vi "WM_CAP - Edit Format.vi"(0 "hwnd":u32, 5 "WM_CAP_START":u32, 11 "Error":errorcluster) -> (15 "error out":errorcluster)   [LabVIEW 2022 SP3]
uses:
  user32.dll
panel:
  in  "Apply":bool
  in  "Compression":string
  in  "BitCount":i16=24
  in  "Height":i32=480
  in  "Width":i32=640
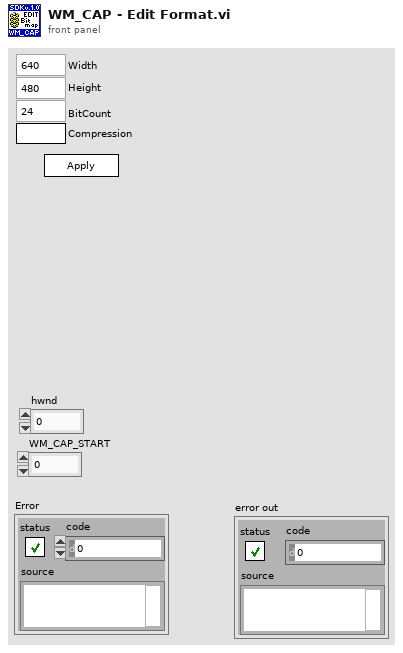
[diagram p1: front panel]
types:
  T1 = cluster{"biSize":i32, "biWidth":i32, "biHeight":i32, "biPlanes":i16, "biBitCount":i16, "biCompression":i32, "biSizeImage":i32, "biXPelsPerMeter":i32, "biYPelsPerMeter":i32, "biClrUsed":i32, "biClrImportant":i32, "Colors":u32[]}
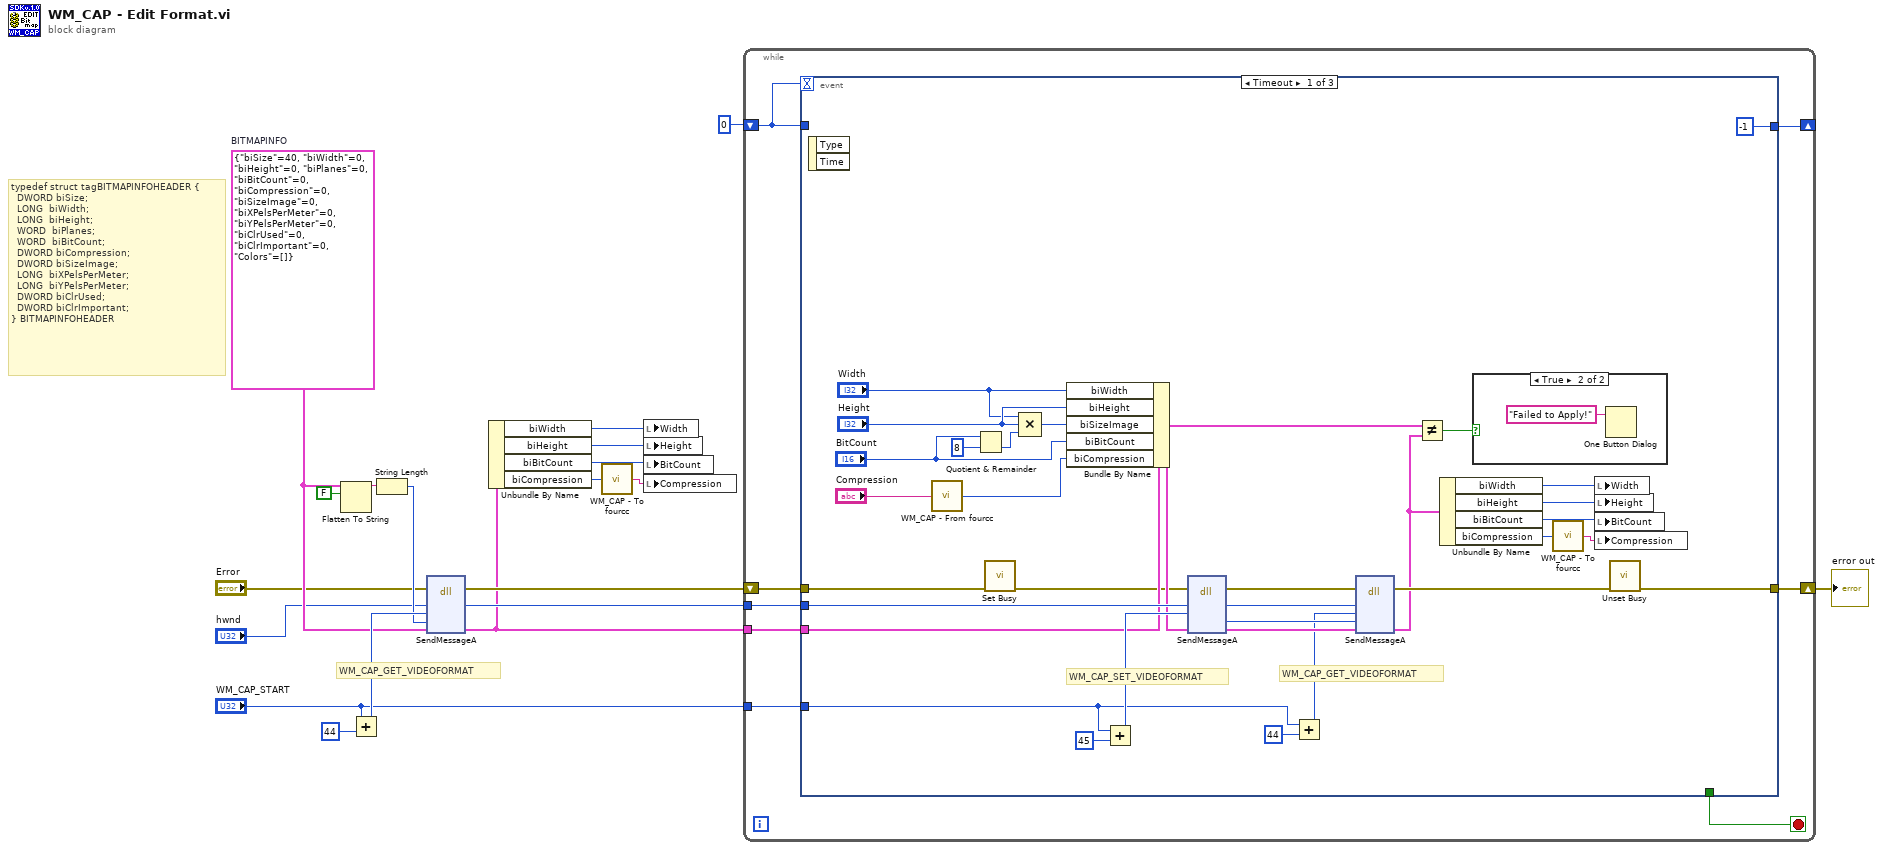
[diagram p0: block diagram]
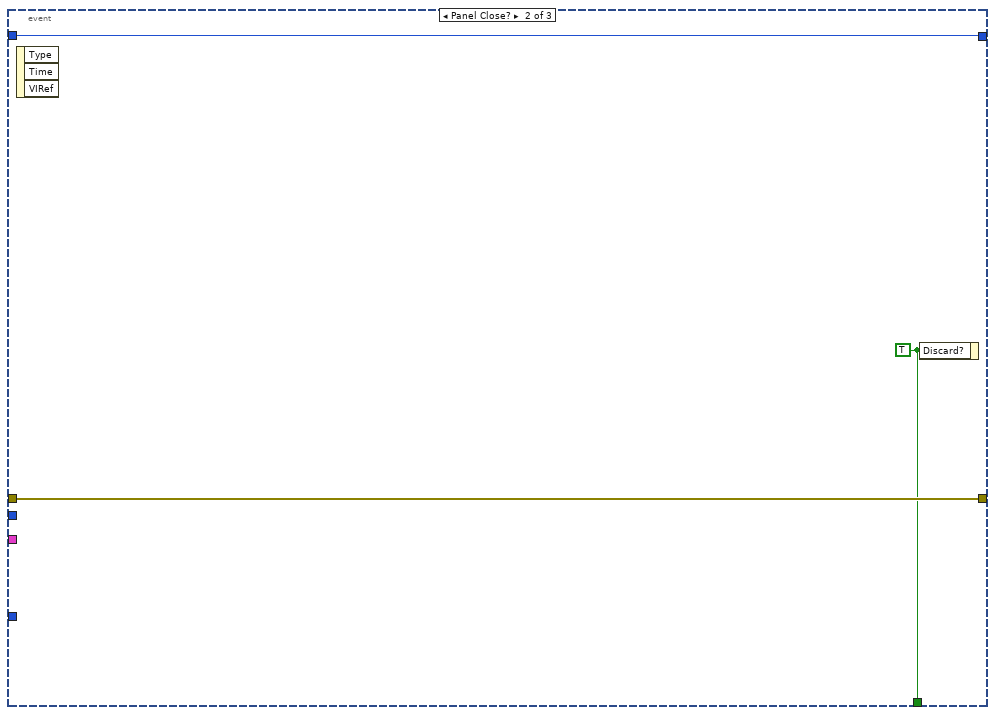
[diagram p3: hidden frame]
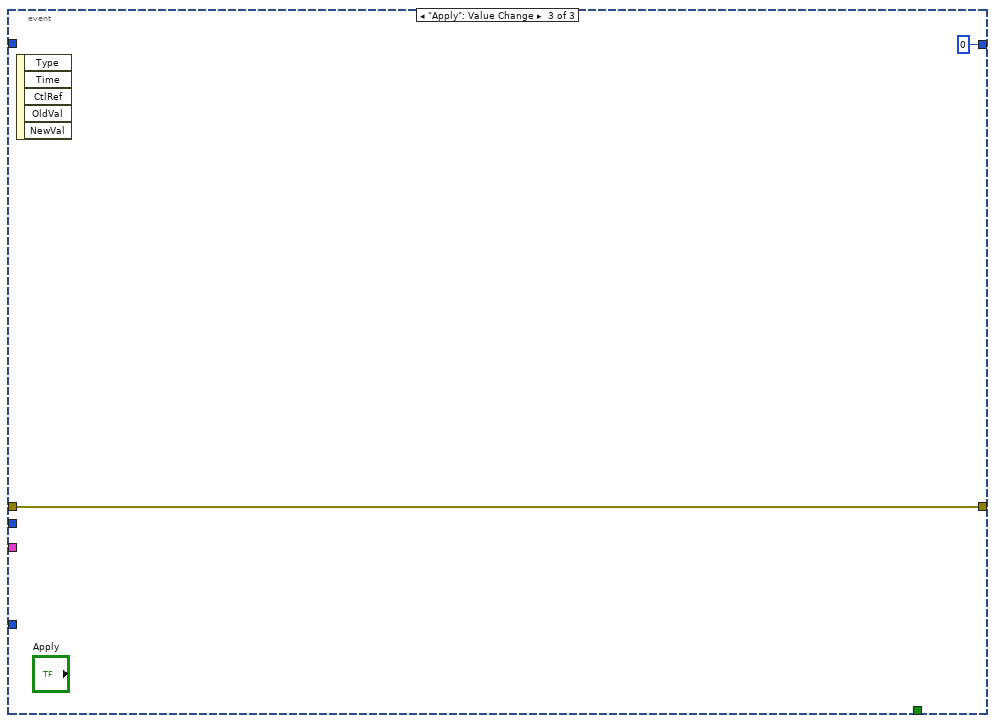
[diagram p4: hidden frame]
diagram:
  w12 = T1 {"biSize"=40, "biWidth"=0, "biHeight"=0, "biPlanes"=0, "biBitCount"=0, "biCompression"=0, "biSizeImage"=0, "biXPelsPerMeter"=0, "biYPelsPerMeter"=0, "biClrUsed"=0, "biClrImportant"=0, "Colors"=[]}  # BITMAPINFO
  # "typedef struct tagBITMAPINFOHEADER {\n  DWORD biSize;\n  LONG  biWidth;\n  LONG  biHeight;\n  WORD  biPlanes;\n  WORD  biBitCount;\n  DWORD biCompression;\n  DWORD biSizeImage;\n  LONG  biXPelsPerMeter;\n  LONG  biYPelsPerMeter;\n  DWORD biClrUsed;\n  DWORD biClrImportant;\n} BITMAPINFOHEADER"
  # "WM_CAP_GET_VIDEOFORMAT"
  n1 = Flatten To String(anything=w12, prepend array or string size? (T)=FALSE) -> (data string=w14:string)  [unwired: 2 in, 2 out]
  n2 = Add(x="WM_CAP_START", y=u16 44) -> (x+y=w17:u32)
  n3 = String Length(string=w14) -> (length=w16:i32)
  n4 = dll-call lib="user32.dll" fn="SendMessageA"(error in="Error", "hwnd"="hwnd", "msg"=w17, "wParam"=w16, "lparam"=w12) -> (error out=w9:errorcluster, "hwnd"=w7:u32, "lparam"=w6:T1)  [unwired: 5 in, 1 out]
  n5 = Unbundle By Name(w6) -> ("biWidth"=w5:i32, "biHeight"=w4:i32, "biBitCount"=w3:i16, "biCompression"=w2:i32)
  n6 = call "WM_CAP - To fourcc.vi"("biCompression"=w2) -> ("FOURCC"=w1:string)  [unwired: 14 in]
  n7 = local write "Width"(w5) -> ()
  n8 = local write "Height"(w4) -> ()
  n9 = local write "BitCount"(w3) -> ()
  n10 = local write "Compression"(w1) -> ()
  n11 = while {
    tunnel: w7 -> [w25]
    tunnel: "WM_CAP_START" -> [w24]
    shift-right: [w23] -> _
    shift-left: 0 -> [w21]
    shift-right: [w27] -> w19
    shift-left: w9 -> [w26]
    tunnel: w6 -> [w20]
    stop <- w22 stop-if-true
    n12 = event shown="[0] Timeout" {
      selector: _ -> [_ _ _]
      dyn-events: _ -> [_ _ _]
      timeout: w21 -> [_ _ _]
      tunnel: [w28 w63 w65] -> w27
      tunnel: w26 -> [w45 w63 w65]
      tunnel: w25 -> [w44 _ _]
      tunnel: w24 -> [w41 _ _]
      tunnel: [-1 w61 0] -> w23
      tunnel: [_ w62 _] -> w22
      tunnel: w21 -> [_ w61 _]
      tunnel: w20 -> [w43 _ _]
      event Timeout {
        # "WM_CAP_GET_VIDEOFORMAT"
        # "WM_CAP_SET_VIDEOFORMAT"
        n13 = event-data() -> ()  [unwired: 1 in, 2 out]
        n14 = call "WM_CAP - From fourcc.vi"("FOURCC"="Compression") -> ("biCompression"=w33:i32)  [unwired: 14 in]
        n15 = Quotient & Remainder(x="BitCount", y=u16 8) -> (floor(x/y)=w49:u16)  [unwired: 1 out]
        n16 = call <vilib>:"Set Busy.vi"("error in (no error)"=w45) -> ("error out"=w29:errorcluster)  [unwired: 9 in, 1 out]
        n17 = Compound Arithmetic op=MULTIPLY("Width", "Height", w49) -> (w51:i32)
        n18 = Bundle By Name(cluster=w43, "biWidth"="Width", "biHeight"="Height", "biSizeImage"=w51, "biBitCount"="BitCount", "biCompression"=w33) -> (w31:T1)
        n19 = Add(x=w41, y=u16 45) -> (x+y=w58:u32)
        n20 = dll-call lib="user32.dll" fn="SendMessageA"(error in=w29, "hwnd"=w44, "msg"=w58, "lparam"=w31) -> (error out=w57:errorcluster, "hwnd"=w56:u32, "wParam"=w55:u32, "lparam"=w54:T1)  [unwired: 5 in, 1 out]
        n21 = Add(x=w41, y=u16 44) -> (x+y=w40:u32)
        n22 = dll-call lib="user32.dll" fn="SendMessageA"(error in=w57, "hwnd"=w56, "msg"=w40, "wParam"=w55, w54) -> (error out=w47:errorcluster, w32:T1)  [unwired: 6 in, 1 out]
        n23 = Not Equal?(x=w31, y=w32) -> (x != y?=w30:bool)
        n24 = Unbundle By Name(w32) -> ("biWidth"=w35:i32, "biHeight"=w36:i32, "biBitCount"=w37:i16, "biCompression"=w38:i32)
        n25 = case shown="True" w30 {
          frame False {
          }
          frame True {
            n26 = One Button Dialog(message="Failed to Apply!") -> ()  [unwired: 1 in, 1 out]
          }
        }
        n27 = call "WM_CAP - To fourcc.vi"("biCompression"=w38) -> ("FOURCC"=w39:string)  [unwired: 14 in]
        n28 = local write "Width"(w35) -> ()
        n29 = local write "Height"(w36) -> ()
        n30 = local write "BitCount"(w37) -> ()
        n31 = local write "Compression"(w39) -> ()
        n32 = call <vilib>:"Unset Busy.vi"("error in (no error)"=w47) -> ("error out"=w28:errorcluster)  [unwired: 10 in]
      }
      event Panel Close? {
        w62 = TRUE ("Discard?")
        n33 = event-data() -> ()  [unwired: 1 in, 3 out]
        n34 = event-data("Discard?"=w62) -> ()  [unwired: 1 in, 1 out]
      }
      event "Apply": Value Change {
        n35 = event-data() -> ()  [unwired: 1 in, 5 out]
      }
    }
  }
  "error out" <- w19
